vi "Configure Event Timing Measurement Dialog.vi"(7 "measurement to be edited":i32, 8 "error in (no error)":errorcluster, 9 "windows":T2[](array[typedef]), 10 "measurements in":T3[](array[typedef]), 11 "Item Ref in":T4 format="%.0x") -> (0 "error out":errorcluster, 2 "measurements out":T3[](array[typedef]), 3 "Item Ref out":T4 format="%.0x")   [LabVIEW 2013, in "Engine Simulation Toolkit System Explorer.lvlib"]
uses:
  Engine Simulation Toolkit System Explorer.lvlib
  Polarity.ctl
  Event Timing Measurement.ctl
  <vilib>/NI Veristand/Custom Device API/Custom Device Item Ref.ctl
  Event Timing Window.ctl
  <vilib>/NI Veristand/Custom Device API/Custom Device API.lvlib
panel:
  in  "Polarity":T1=enum."Active high"
  in  "Window":u16(ring)
  in  "Cancel":bool
  in  "OK":bool
  in  "Name":string
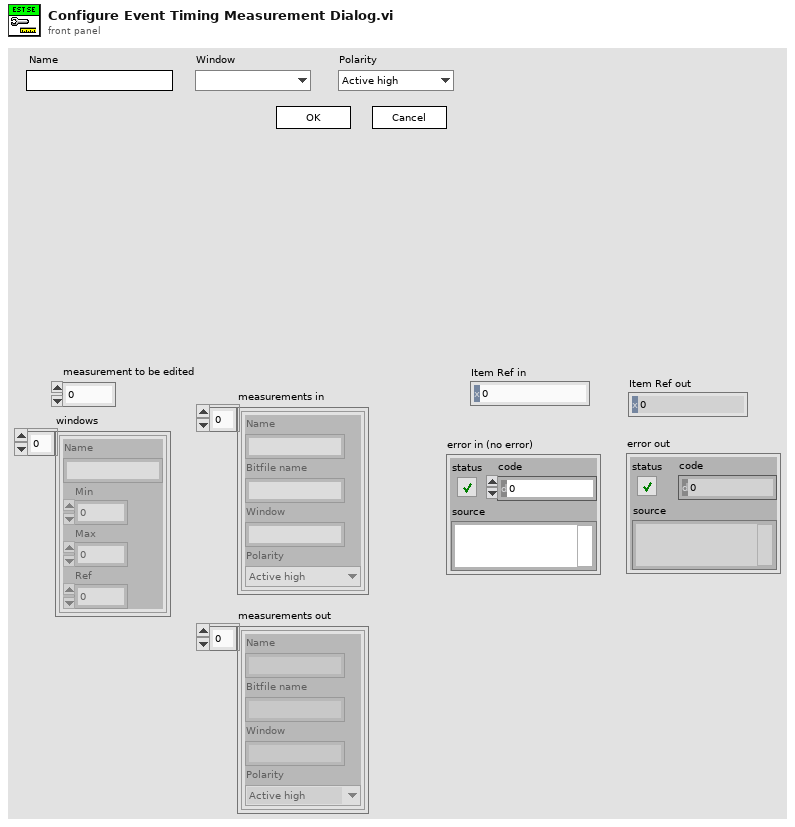
[diagram p1: front panel]
types:
  T1 = typedef "Engine Simulation Toolkit System Explorer.lvlib/Polarity.ctl" = enum16{"Active low", "Active high"}
  T2 = typedef "Engine Simulation Toolkit System Explorer.lvlib/Event Timing Window.ctl" = cluster{"Name":string, "Min":dbl, "Max":dbl, "Ref":dbl}
  T3 = typedef "Engine Simulation Toolkit System Explorer.lvlib/Event Timing Measurement.ctl" = cluster{"Name":string, "Bitfile name":string, "Window":string, "Polarity":T1}
  T4 = typedef "Custom Device API.lvlib/Custom Device Item Ref.ctl" = u64
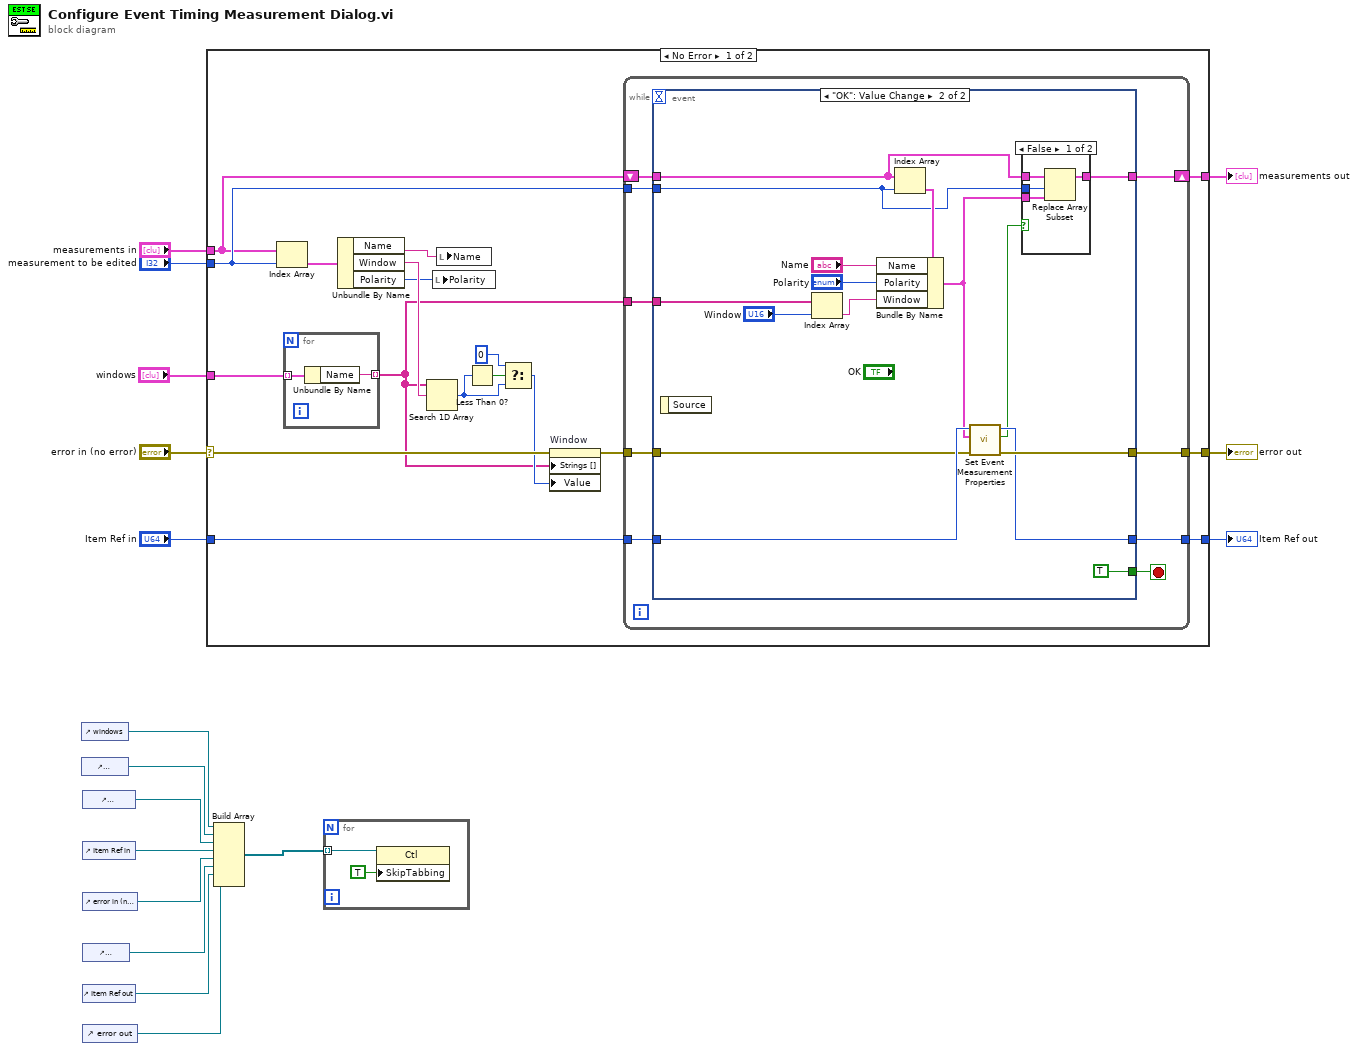
[diagram p0: block diagram]
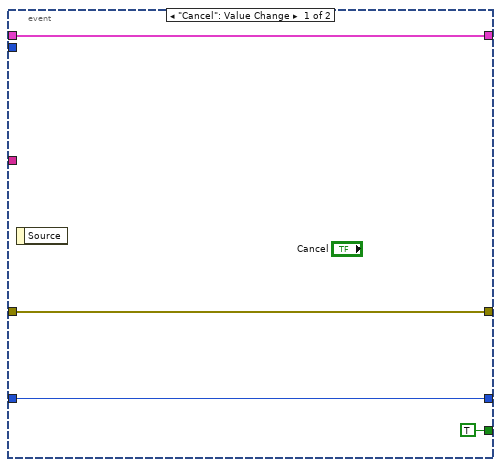
[diagram p2: hidden frame]
diagram:
  n1 = control-ref of="windows"() -> (w4:refnum<vi>)
  n2 = control-ref of="measurements out"() -> (w3:refnum<vi>)
  n3 = control-ref of="measurement to be edited"() -> (w11:refnum<vi>)
  n4 = control-ref of="Item Ref in"() -> (w10:refnum<vi>)
  n5 = control-ref of="error in (no error)"() -> (w9:refnum<vi>)
  n6 = control-ref of="measurements in"() -> (w8:refnum<vi>)
  n7 = control-ref of="Item Ref out"() -> (w2:refnum<vi>)
  n8 = control-ref of="error out"() -> (w1:refnum<vi>)
  n9 = case shown="No Error" "error in (no error)" {
    selector: "error in (no error)" -> [w26 w74]
    tunnel: "measurements in" -> [w33 w73]
    tunnel: "measurement to be edited" -> [w34 _]
    tunnel: [w35 w74] -> w14
    tunnel: [w32 w73] -> w6
    tunnel: "Item Ref in" -> [w31 w72]
    tunnel: [w30 w72] -> w12
    tunnel: "windows" -> [w27 _]
    frame No Error {
      n10 = Index Array(array=w33, index=w34) -> (element=w28:T3)
      n11 = for {
        tunnel: w27 -> [w37] mode=indexing
        tunnel: [w36] -> w18 mode=indexing
        n12 = Unbundle By Name(w37) -> ("Name"=w36:string)
      }
      n13 = Unbundle By Name(w28) -> ("Name"=w29:string, "Window"=w24:string, "Polarity"=w19:T1)
      n14 = Search 1D Array(1D array=w18, element=w24) -> (index of element=w22:i32)  [unwired: 1 in]
      n15 = local write "Polarity"(w19) -> ()
      n16 = local write "Name"(w29) -> ()
      n17 = Less Than 0?(x=w22) -> (x < 0?=w23:bool)
      n18 = Select(t=0, s=w23, f=w22) -> (s? t:f=w20:i32)
      n19 = property on="Window" class="Ring (strict)"(error in=w26, "Strings []"=w18, "Value"=w20) -> (error out=w25:errorcluster)  [unwired: 1 in, 1 out]
      n20 = while {
        tunnel: [w39] -> w35
        tunnel: w25 -> [w46]
        tunnel: w34 -> [w45]
        tunnel: w31 -> [w42]
        tunnel: [w41] -> w30
        tunnel: w18 -> [w38]
        shift-right: [w43] -> w32
        shift-left: w33 -> [w44]
        stop <- w40 stop-if-true
        n21 = event shown="[1] \"OK\": Value Change" {
          selector: _ -> [_ _]
          dyn-events: _ -> [_ _]
          timeout: _ -> [_ _]
          tunnel: [w50 w60] -> w39
          tunnel: w46 -> [w50 w55]
          tunnel: w45 -> [_ w63]
          tunnel: w44 -> [w49 w64]
          tunnel: [w49 w62] -> w43
          tunnel: w42 -> [w48 w59]
          tunnel: [w48 w58] -> w41
          tunnel: [TRUE TRUE] -> w40
          tunnel: w38 -> [_ w61]
          event "Cancel": Value Change {
            n22 = event-data() -> ()  [unwired: 1 in, 1 out]
          }
          event "OK": Value Change {
            n23 = event-data() -> ()  [unwired: 1 in, 1 out]
            n24 = Index Array(array=w61, index="Window") -> (element=w51:string)
            n25 = Index Array(array=w64, index=w63) -> (element=w65:T3)
            n26 = Bundle By Name(cluster=w65, "Name"="Name", "Polarity"="Polarity", "Window"=w51) -> (w57:T3)
            n27 = call "Set Event Measurement Properties.vi"("error in (no error)"=w55, "measurement"=w57, "Item Ref in"=w59) -> ("error out"=w60:errorcluster, "failed"=w56:bool, "Item Ref out"=w58:T4)  [unwired: 6 in]
            n28 = case shown="False" w56 {
              tunnel: w64 -> [w70 w71]
              tunnel: w63 -> [w69 _]
              tunnel: [w68 w71] -> w62
              tunnel: w57 -> [w67 _]
              frame False {
                n29 = Replace Array Subset(array=w70, new element=w67, index=w69) -> (w68:T3[])
              }
              frame True {
              }
            }
          }
        }
      }
    }
    frame Error {
    }
  }
  "error out" <- w14
  "Item Ref out" <- w12
  "measurements out" <- w6
  n30 = Build Array(w4, w3, w11, w10, w9, w8, w2, w1) -> (w7:refnum<vi>[])
  n31 = for {
    tunnel: w7 -> [w76] mode=indexing
    n32 = property class="Ctl"(reference=w76, "SkipTabbing"=TRUE ("Skip When Tabbing")) -> ()  [unwired: 1 in, 2 out]
  }
